vi "Lr5SubVI.vi"(0 "Samples":i32, 1 "Out":bool, 2 "Noise amplitude":dbl(knob) scale=0.0..3.0, 5 "Sine frequency":dbl(slide) scale=0.1..1.0, 7 "Noise":u16(ring) items=["Periodic Random", "Uniform white", "Gaussian white"], 9 "Signal Type":enum16{"sine", "square"}(ring), 12 "Frequency":dbl(knob) scale=0.1..100.0, 13 "Signal amplitude":dbl(slide) scale=1.0..10.0, 14 "Square wave duty cycle(%)":dbl) -> ()   [LabVIEW 2012]
uses:
  <vilib>/Analysis/NI_AALBase.lvlib
  <vilib>/Analysis/NI_AALPro.lvlib
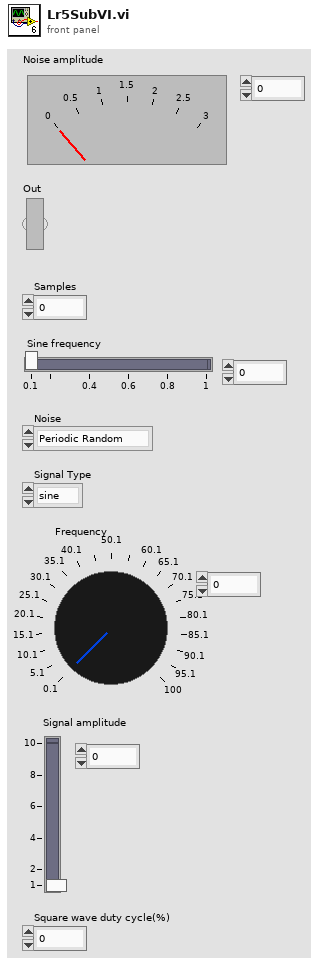
[diagram p1: front panel]
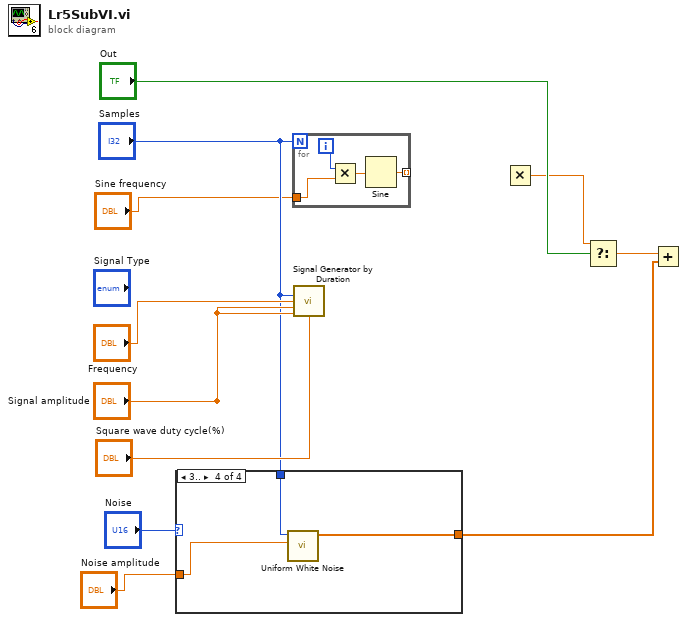
[diagram p0: block diagram]
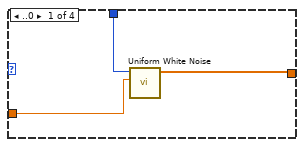
[diagram p2: hidden frame]
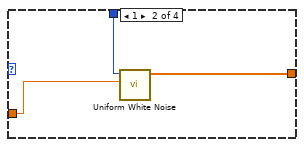
[diagram p3: hidden frame]
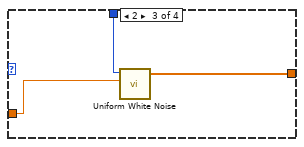
[diagram p4: hidden frame]
diagram:
  n1 = case shown="3.." "Noise" {
    tunnel: "Samples" -> [w15 w19 w21 w24]
    tunnel: [w16 w18 w22 w25] -> w12
    tunnel: "Noise amplitude" -> [w14 w17 w20 w23]
    frame ..0 {
      n2 = call <vilib>:"Uniform White Noise.vi"("amplitude"=w14, "samples"=w15) -> ("uniform white noise"=w16:dbl[])  [unwired: 8 in, 1 out]
    }
    frame 1 {
      n3 = call <vilib>:"Uniform White Noise.vi"("amplitude"=w17, "samples"=w19) -> ("uniform white noise"=w18:dbl[])  [unwired: 8 in, 1 out]
    }
    frame 2 {
      n4 = call <vilib>:"Uniform White Noise.vi"("amplitude"=w20, "samples"=w21) -> ("uniform white noise"=w22:dbl[])  [unwired: 8 in, 1 out]
    }
    frame 3.. {
      n5 = call <vilib>:"Uniform White Noise.vi"("amplitude"=w23, "samples"=w24) -> ("uniform white noise"=w25:dbl[])  [unwired: 8 in, 1 out]
    }
  }
  n6 = for {
    N: "Samples" -> [_]
    tunnel: "Sine frequency" -> [w27]
    tunnel: [w26] -> _ mode=indexing
    i -> [w28]
    n7 = Multiply(x=w28, y=w27) -> (x*y=w29:dbl)
    n8 = Sine(x=w29) -> (sin(x)=w26:dbl)
  }
  n9 = call <vilib>:"Signal Generator by Duration.vi"("# of samples"="Samples", "frequency"="Frequency", "amplitude"="Signal amplitude", "dc offset"="Signal amplitude", "square wave duty cycle (%)"="Square wave duty cycle(%)") -> ("signal"=w7:dbl[])  [unwired: 7 in, 3 out]
  n10 = Multiply() -> (x*y=w9:dbl)  [unwired: 2 in]
  n11 = Select(t=w9, s="Out") -> (f=w8:dbl, s? t:f=w11:dbl)
  n12 = Add(x=w11, y=w12) -> ()  [unwired: 1 out]
